vi "Init Save Image Class.vi"(8 "error in (no error)":errorcluster, 11 "Image Constructor in":refnum<class "Image Constructor.lvclass">) -> (0 "error out":errorcluster, 3 "Image Constructor out":refnum<class "Image Constructor.lvclass">)   [LabVIEW 2018, in "Image Constructor.lvclass"]
uses:
  Image Constructor.lvclass
  Save Image/Save Image.lvclass
  Header/Header.lvclass
panel:
  in  "Header.lvclass":refnum<class "Header.lvclass">
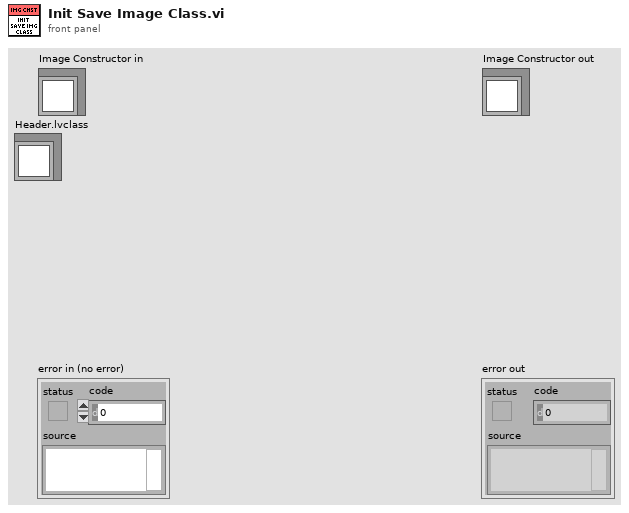
[diagram p1: front panel]
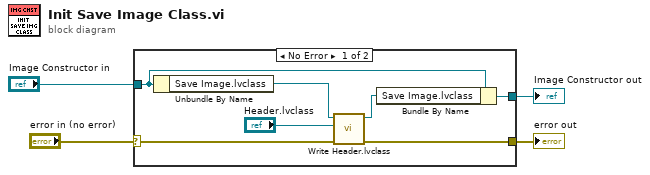
[diagram p0: block diagram]
diagram:
  n1 = case shown="No Error" "error in (no error)" {
    selector: "error in (no error)" -> [w6 w13]
    tunnel: [w7 w13] -> w3
    tunnel: [w11 w12] -> w1
    tunnel: "Image Constructor in" -> [w10 w12]
    frame No Error {
      n2 = Unbundle By Name(w10) -> ("Save Image.lvclass"=w8:refnum<class "Save Image.lvclass">)
      n3 = call "Write Header.lvclass.vi"("error in (no error)"=w6, "Header.lvclass"="Header.lvclass", "Save Image in"=w8) -> ("error out"=w7:errorcluster, "Save Image out"=w9:refnum<class "Save Image.lvclass">)  [unwired: 7 in]
      n4 = Bundle By Name(cluster=w10, "Save Image.lvclass"=w9) -> (w11:refnum<class "Image Constructor.lvclass">)
    }
    frame Error {
    }
  }
  "error out" <- w3
  "Image Constructor out" <- w1
